vi "Configure IQ Source Ratio.vi"(8 "error in (no error)":errorcluster, 10 "Source Ratio (0 dB)":dbl, 11 "VISA resource name":refnum<visa-resource-name>) -> (0 "error out":errorcluster, 3 "VISA resource name out":refnum<visa-resource-name>)   [LabVIEW 2014, in "Agilent PSG MXG Series.lvlib"]
doc: "Sets the power level difference (ratio) between the source one and source two signals when the two signals are summed together.\n\n<B>Notes:</B>\n(1) This VI is valid only in N5172B and N5182B."
uses:
  Agilent PSG MXG Series.lvlib
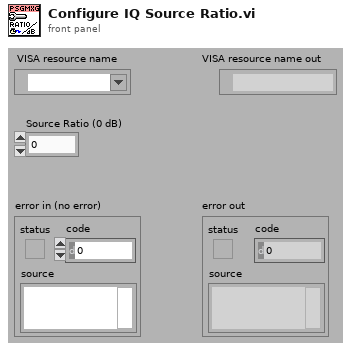
[diagram p1: front panel]
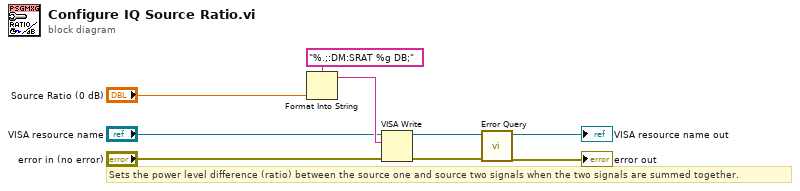
[diagram p0: block diagram]
diagram:
  # "Sets the power level difference (ratio) between the source one and source two signals when the two signals are summed together."
  n1 = Format Into String(format string="%.;:DM:SRAT %g DB;", "Source Ratio (0 dB)") -> (resulting string=w7:string)  [unwired: 2 in, 1 out]
  n2 = VISA Write(VISA resource name="VISA resource name", write buffer=w7, error in (no error)="error in (no error)") -> (VISA resource name out=w4:refnum<visa-resource-name>, error out=w3:errorcluster)  [unwired: 1 out]
  n3 = call "Error Query.vi"("error in (no error)"=w3, "VISA resource name"=w4) -> ("error out"=→"error out":errorcluster, "VISA resource name out"=→"VISA resource name out":refnum<visa-resource-name>)  [unwired: 8 out]
